vi "Play Sound.vi"(8 "error in (no error)":errorcluster, 11 "Sound Name":string) -> (0 "error out":errorcluster)   [LabVIEW 2015, in "Resource Manager.lvclass"]
uses:
  Resource Manager.lvclass
  Resource Manager.lvclass/Resource Manager.ctl
  Globals.vi
  LabSDL2/Source/Libraries/LibSDL2_Mixer Wrapper/LibSDL2_Mixer.lvlib
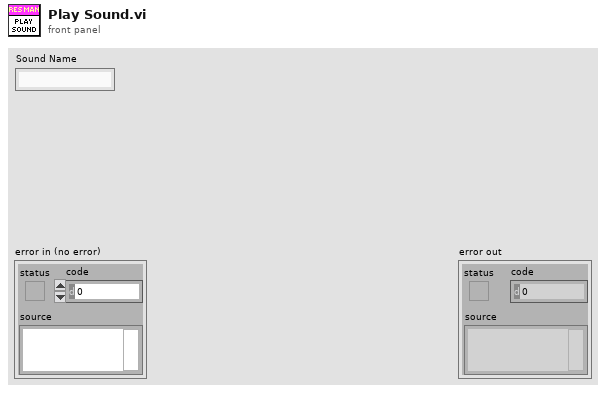
[diagram p1: front panel]
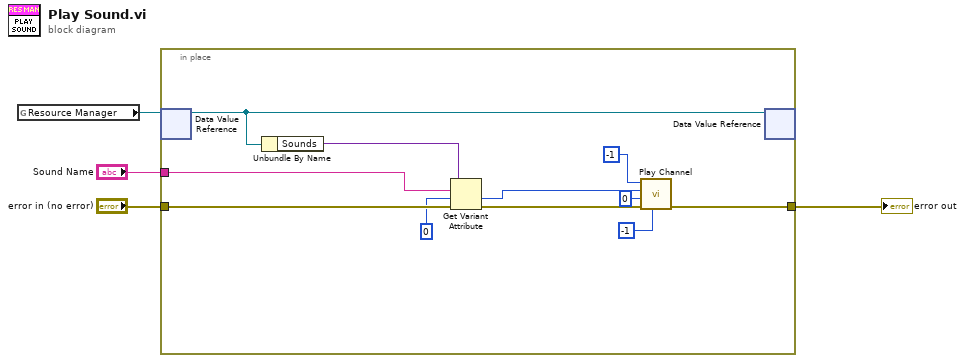
[diagram p0: block diagram]
diagram:
  n1 = global read "Globals.vi" "Resource Manager"() -> (w1:refnum<data-value>)
  n2 = in-place {
    in-place-border: "error in (no error)" -> [w14]
    in-place-border: [w7] -> w3
    in-place-border: "Sound Name" -> [w13]
    n3 = in-place-dvr #1(w1) -> (w6:refnum<class "Resource Manager.lvclass">)  [unwired: 1 out]
    n4 = Unbundle By Name(w6) -> ("Sounds"=w15:variant)
    n5 = Get Variant Attribute(Variant=w15, name=w13, default value (empty Variant)=u32 0 ("Chunk Pointer"), error in=w14) -> (value=w5:u32, error out=w8:errorcluster)  [unwired: 2 out]
    n6 = call "Play Channel.vi"("Ticks"=-1, "error in"=w8, "Loops"=0, "Chunk Pointer"=w5, "Channel"=-1) -> ("error out"=w7:errorcluster)  [unwired: 5 in, 1 out]
    n7 = in-place-dvr #1(w6) -> ()  [unwired: 2 out]
  }
  "error out" <- w3
